vi "digitalOutTest.vi"() -> ()   [LabVIEW 2017]
uses:
  <vilib>/DAQmx/read.llb/DAQmx Read (Analog 2D DBL NChan NSamp).vi
  <vilib>/DAQmx/write.llb/DAQmx Write (Digital 2D U8 NChan NSamp).vi
  <vilib>/DAQmx/create/channels.llb/DAQmx Create Channel (DO-Digital Output).vi
  <vilib>/Waveform/DWDTOps.llb/DWDT Boolean Array to Digital.vi
  <vilib>/Waveform/DWDTOps.llb/DWDT Digital to Binary U8.vi
  <vilib>/DAQmx/configure/timing.llb/DAQmx Timing (Sample Clock).vi
  <vilib>/DAQmx/miscellaneous.llb/DAQmx Fill In Error Info.vi
  <vilib>/DAQmx/create/channels.llb/DAQmx Create Channel (AI-Voltage-Basic).vi
  <vilib>/DAQmx/configure/trigger.llb/DAQmx Reference Trigger (Analog Edge).vi
panel:
  out "Waveform Graph":dbl[][](graph)
  in  "rate":dbl=1000.0 format="%0.2f"
  in  "samples per channel":i32=1000
  out "number of samples written per channel":u32
  out "x-y":u32
  out "Digital Waveform Graph":digitalwaveform(graph)
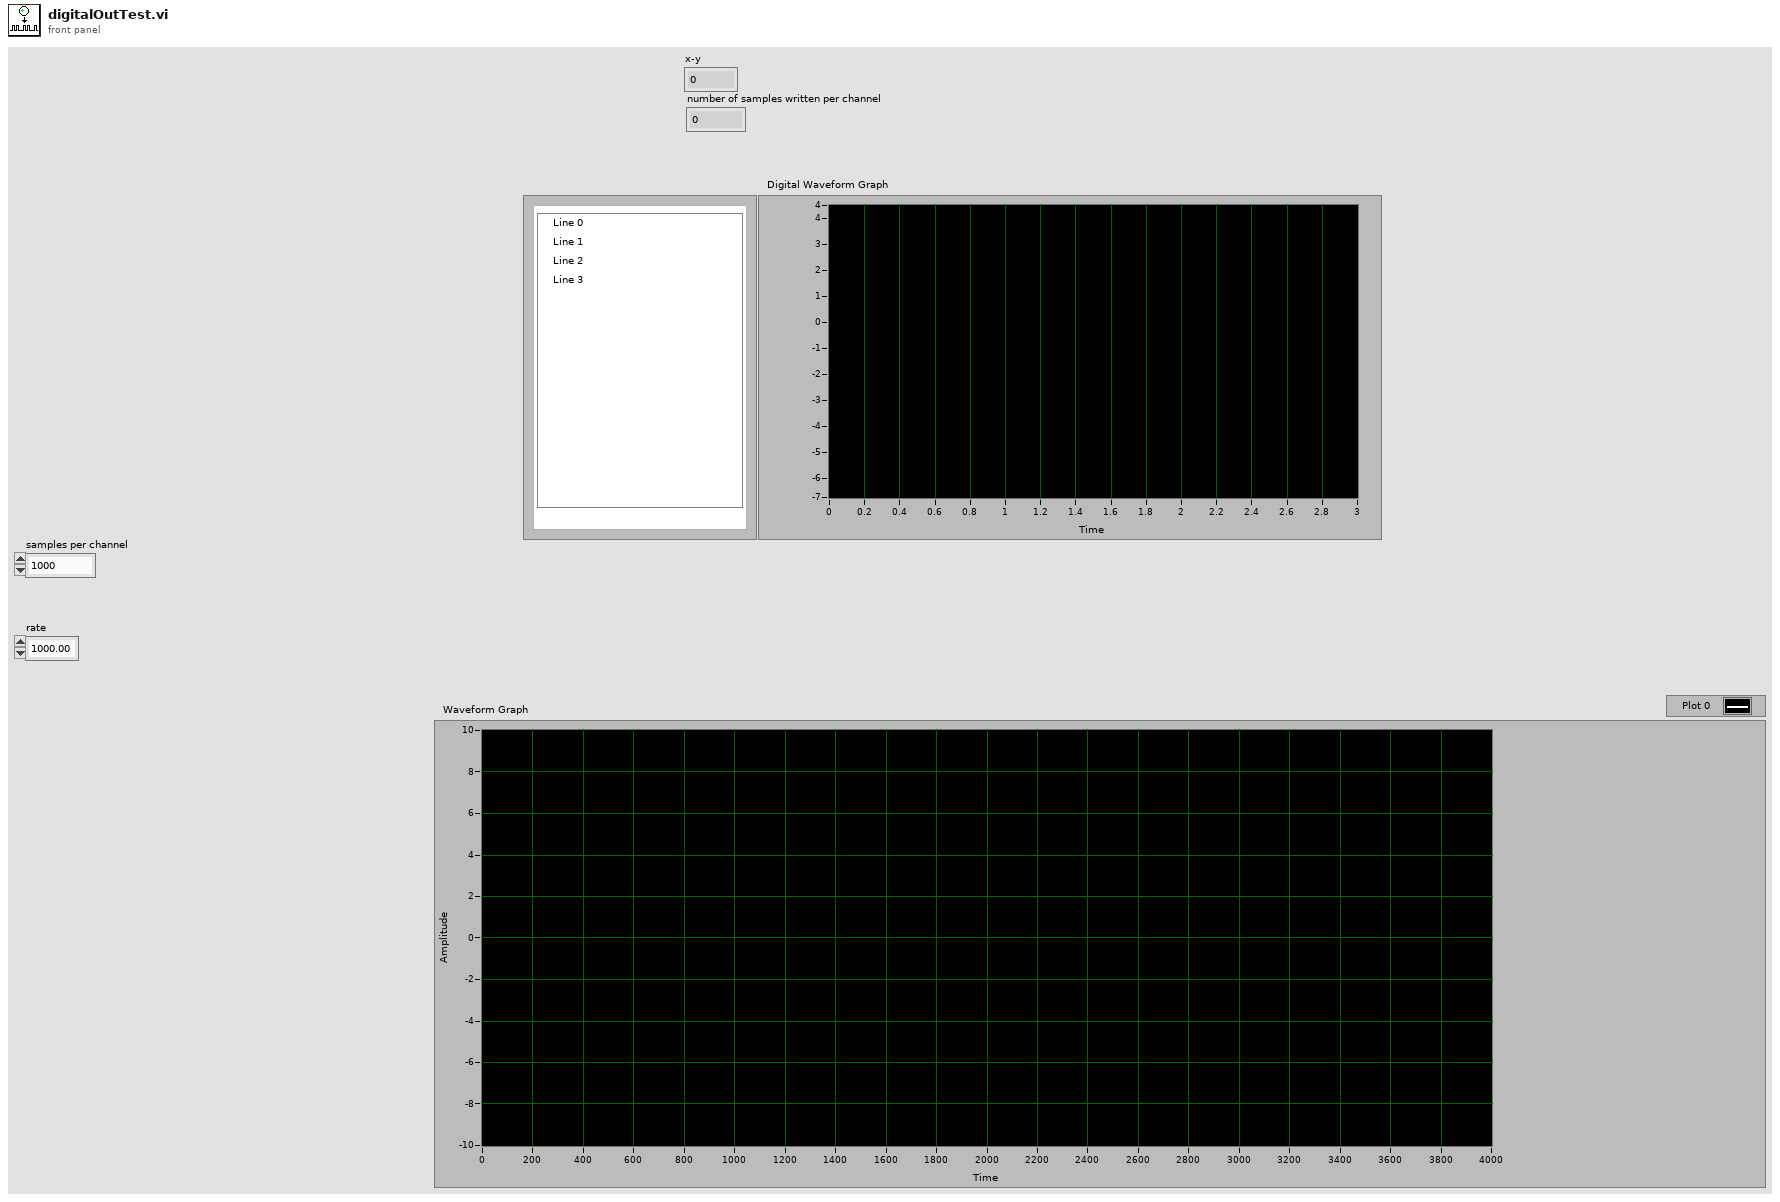
[diagram p1: front panel]
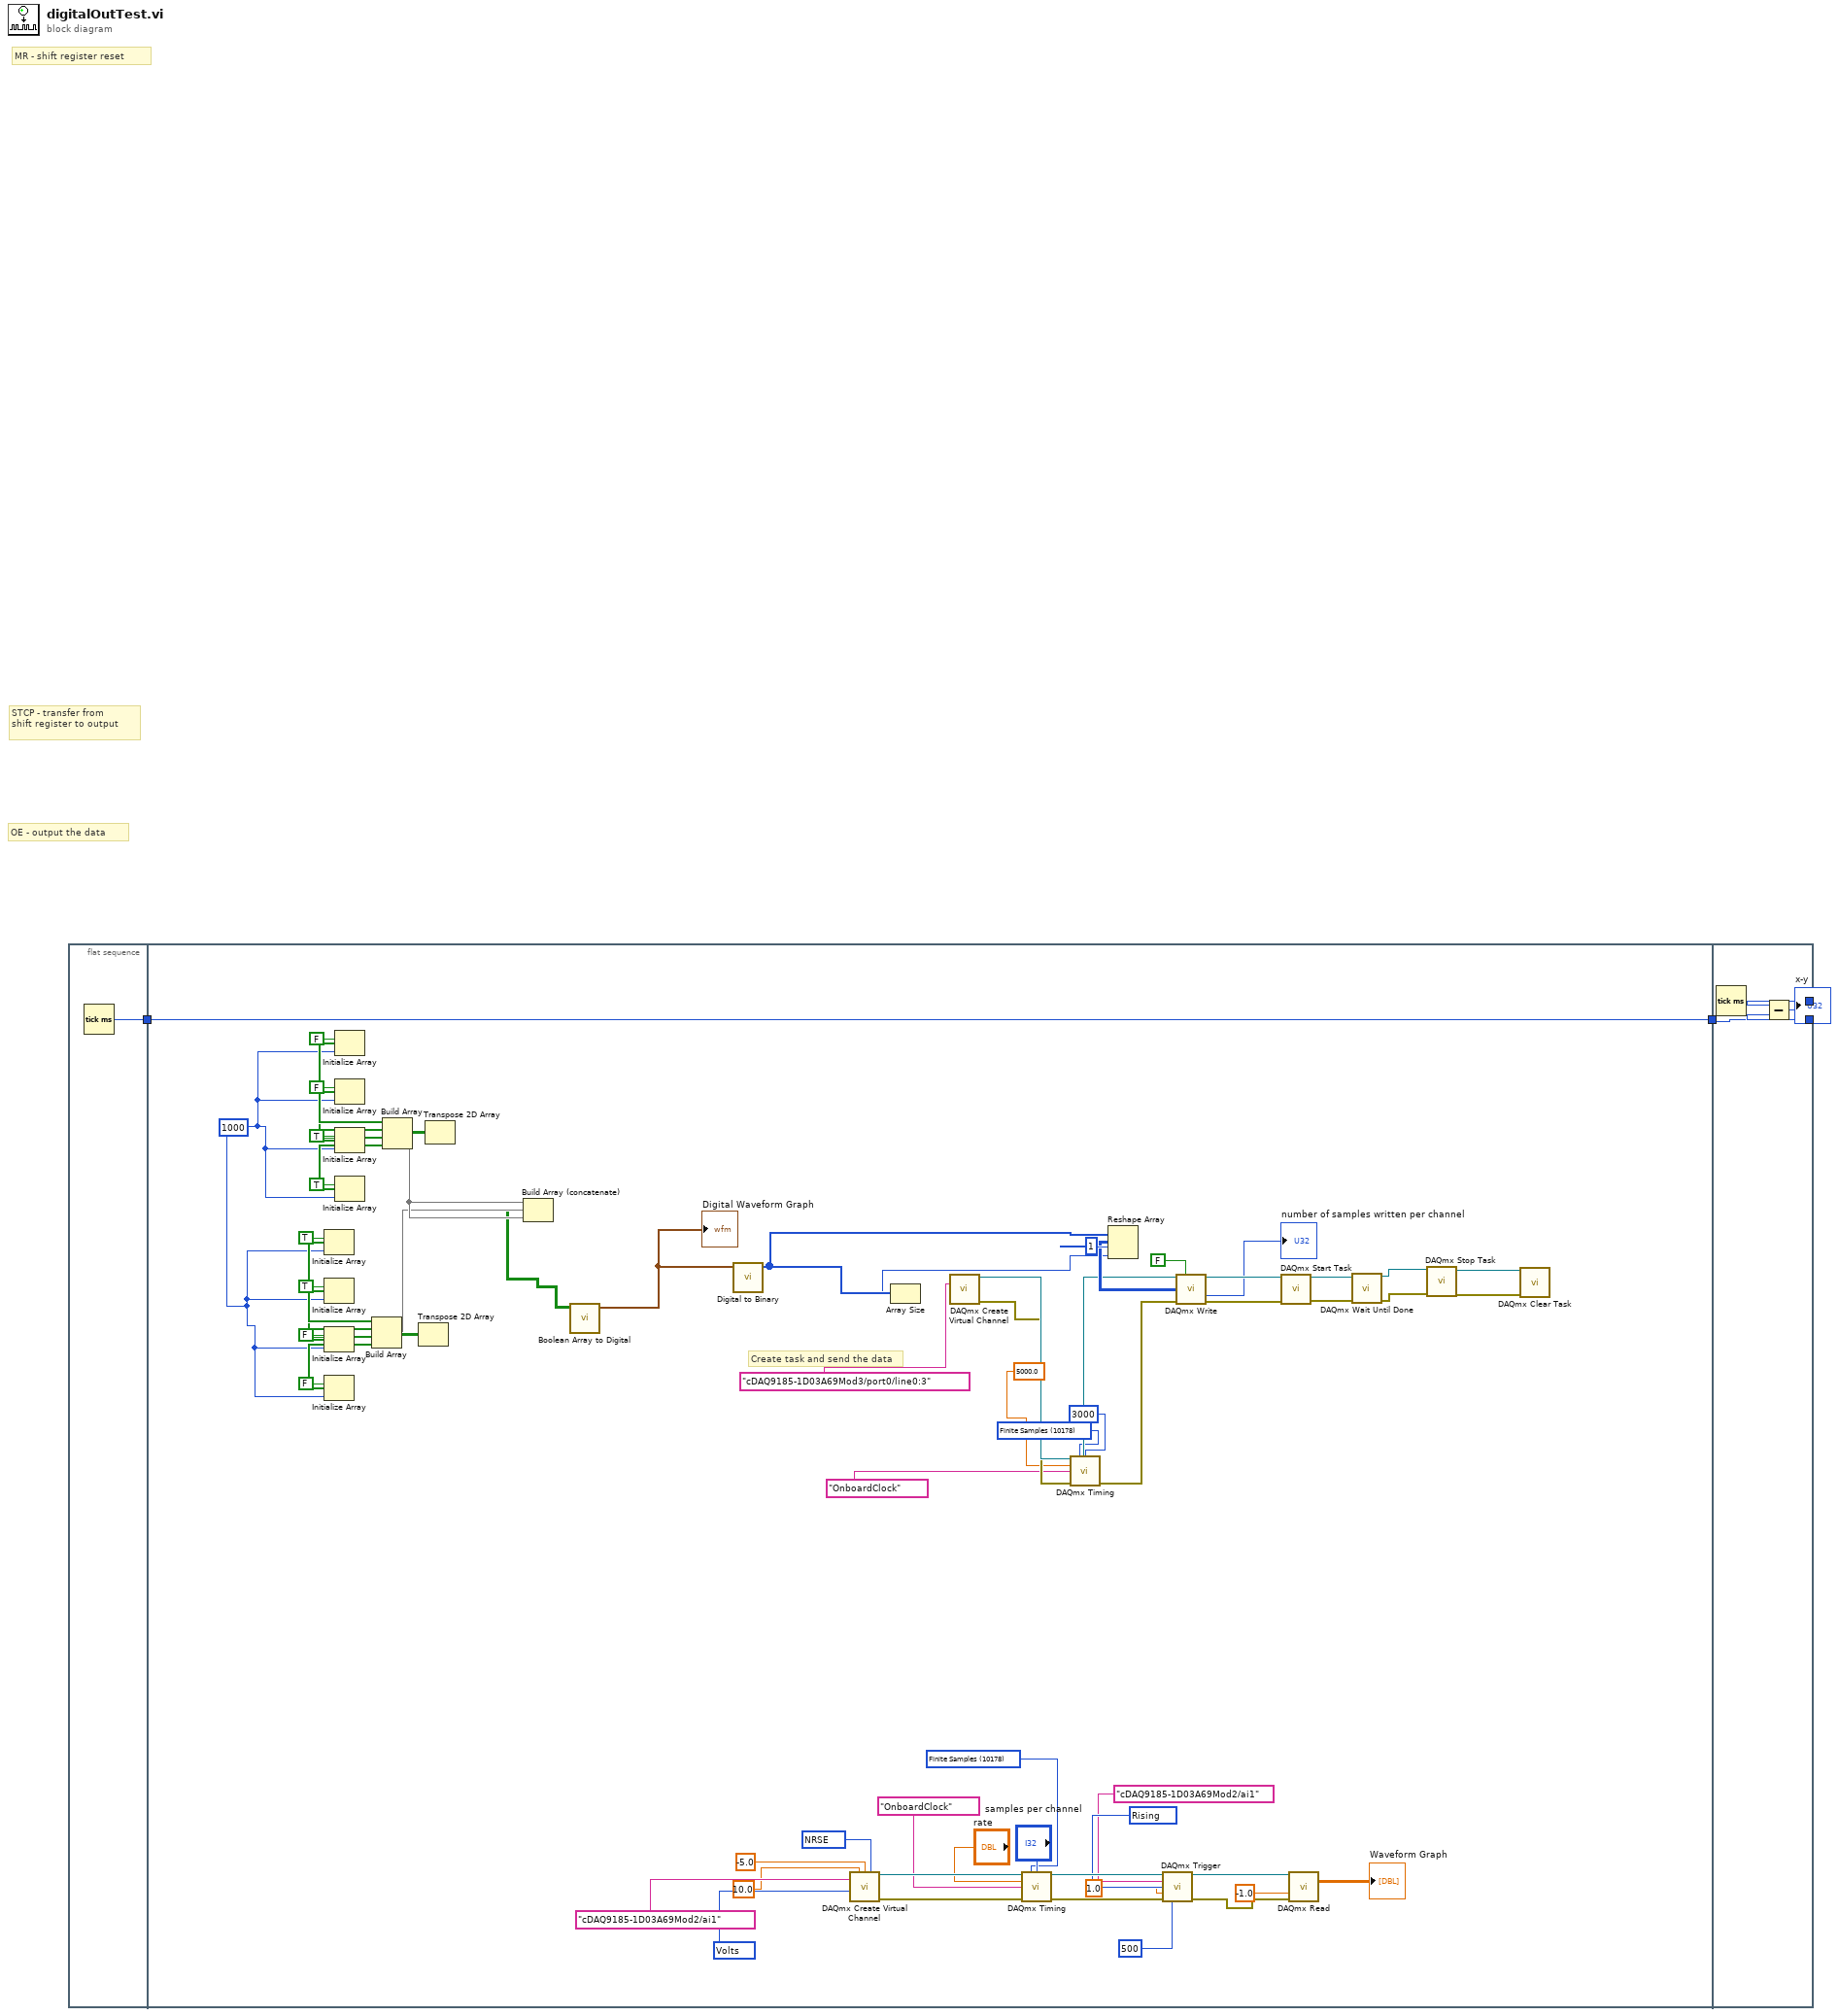
[diagram p0: block diagram]
diagram:
  # "OE - output the data"
  # "STCP - transfer from \nshift register to output"
  # "MR - shift register reset"
  n1 = flat-sequence {
    tunnel: [w6] -> w2
    tunnel: [w58] -> w3
    tunnel: w2 -> [w58]
    tunnel: [w76] -> w5
    tunnel: [w75] -> w4
    tunnel: w3 -> [w75]
    frame #0 {
      n2 = Tick Count (ms)() -> (millisecond timer value=w6:u32)
    }
    frame #1 {
      w27 = 10178 items=["Finite Samples"=10178, "Continuous Samples"=10123, "Hardware Timed Single Point"=12522] ("sample mode")
      w23 = 10078 items=["Default"=-1, "RSE"=10083, "NRSE"=10078, "Differential"=10106, "Pseudodifferential"=12529] ("input terminal configuration")
      w18 = 10348 items=["Volts"=10348, "From Custom Scale"=10065] ("units")
      w19 = 10280 items=["Rising"=10280, "Falling"=10171] ("edge")
      w33 = 10178 items=["Finite Samples"=10178, "Continuous Samples"=10123, "Hardware Timed Single Point"=12522] ("sample mode")
      w47 = 1000
      # "Create task and send the data"
      n3 = Initialize Array(TRUE, w47) -> (w53:bool[])
      n4 = Initialize Array(TRUE, w47) -> (w52:bool[])
      n5 = Initialize Array(FALSE, w47) -> (w48:bool[])
      n6 = Initialize Array(FALSE, w47) -> (w49:bool[])
      n7 = Initialize Array(FALSE, w47) -> (w64:bool[])
      n8 = Initialize Array(FALSE, w47) -> (w63:bool[])
      n9 = Initialize Array(TRUE, w47) -> (w59:bool[])
      n10 = Initialize Array(TRUE, w47) -> (w60:bool[])
      n11 = Build Array(w53, w52, w48, w49) -> (w44:bool[][])
      n12 = Build Array(w64, w63, w59, w60) -> (w46:bool[][])
      n13 = Transpose 2D Array(2D array=w44) -> (transposed array=w43:bool[][])
      n14 = Transpose 2D Array(2D array=w46) -> (transposed array=w45:bool[][])
      n15 = Build Array (concatenate)(w45, w43, w45) -> (w42:bool[][])
      n16 = call-poly <vilib>:"Boolean Array to Digital.vi"("boolean array"=w42) -> ("digital waveform"=w73:digitalwaveform)  [unwired: 9 in, 1 out]
      "Digital Waveform Graph" <- w73
      n17 = call-poly <vilib>:"Digital to Binary.vi"("digital waveform"=w73) -> ("binary array"=w70:u8[])  [unwired: 9 in, 1 out]
      n18 = call-poly <vilib>:"DAQmx Create Virtual Channel.vi"("maximum value"=10.0, "minimum value"=-5.0, "input terminal configuration"=w23, "physical channels"=tag "cDAQ9185-1D03A69Mod2/ai1", "units"=w18) -> ("task out"=w29:refnum<k21>, "error out"=w30:errorcluster)  [unwired: 9 in]
      n19 = Array Size(array=w70) -> (size(s)=w69:i32)
      n20 = call-poly <vilib>:"DAQmx Create Virtual Channel.vi"("lines"=tag "cDAQ9185-1D03A69Mod3/port0/line0:3") -> ("task out"=w40:refnum<k21>, "error out"=w39:errorcluster)  [unwired: 13 in]
      n21 = call-poly <vilib>:"DAQmx Timing.vi"("task/channels in"=w29, "sample mode"=w27, "samples per channel"="samples per channel", "rate"="rate", "source"=tag "OnboardClock", "error in"=w30) -> ("task out"=w21:refnum<k21>, "error out"=w12:errorcluster)  [unwired: 8 in]
      n22 = call-poly <vilib>:"DAQmx Timing.vi"("task/channels in"=w40, "sample mode"=w33, "samples per channel"=3000, "rate"=5000.0, "source"=tag "OnboardClock", "error in"=w39) -> ("task out"=w41:refnum<k21>, "error out"=w38:errorcluster)  [unwired: 8 in]
      n23 = Reshape Array(w70, 1, w69) -> (w71:u8[][])
      n24 = call-poly <vilib>:"DAQmx Trigger.vi"("task/channels in"=w21, "source"="cDAQ9185-1D03A69Mod2/ai1", "slope"=w19, "level"=1.0, "error in"=w12, "pretrigger samples per channel"=u32 500) -> ("task out"=w20:refnum<k21>, "error out"=w11:errorcluster)  [unwired: 8 in]
      n25 = call-poly <vilib>:"DAQmx Write.vi"("task/channels in"=w41, "auto start"=FALSE, "data"=w71, "error in"=w38) -> ("task out"=w68:refnum<k21>, "number of samples written per channel"=→"number of samples written per channel":u32, "error out"=w67:errorcluster)  [unwired: 9 in]
      n26 = call <vilib>:"DAQmx Start Task.vi"("task/channels in"=w68, "error in"=w67) -> ("task out"=w10:refnum<k21>, "error out"=w7:errorcluster)  [unwired: 12 in]
      n27 = call-poly <vilib>:"DAQmx Read.vi"("task/channels in"=w20, "timeout"=-1.0, "error in"=w11) -> ("data"=→"Waveform Graph":dbl[][])  [unwired: 10 in, 2 out]
      n28 = call <vilib>:"DAQmx Wait Until Done.vi"("task/channels in"=w10, "error in"=w7) -> ("task out"=w9:refnum<k21>, "error out"=w8:errorcluster)  [unwired: 12 in]
      n29 = call <vilib>:"DAQmx Stop Task.vi"("task/channels in"=w9, "error in"=w8) -> ("task out"=w35:refnum<k21>, "error out"=w36:errorcluster)  [unwired: 12 in]
      n30 = call <vilib>:"DAQmx Clear Task.vi"("task in"=w35, "error in"=w36) -> ()  [unwired: 13 in, 1 out]
    }
    frame #2 {
      n31 = Tick Count (ms)() -> (millisecond timer value=w76:u32)
    }
  }
  n32 = Subtract(x=w5, y=w4) -> (x-y=→"x-y":u32)
